vi "ParameterEditor_new.vi"(1 "Previous Parameters":T1=[{"Status"="ADC", "Name"="state (0,1,2)", "Value"=0.0, "Changed"=FALSE}, {"Status"="Camera", "Name"="state (0,1)", "Value"=0.0, "Changed"=FALSE}, {"Status"="Slave", "Name"="state (0,1)", "Value"=0.0, "Changed"=FALSE}, {"Status"="Wait", "Name"="inbit (0...7)", "Value"=0.0, "Changed"=FALSE}, {"Status"="e-", "Name"="enable (0,1)", "Value"=0.0, "Changed"=FALSE}, {"Status"="e-", "Name"="burn time (s)", "Value"=0.0, "Changed"=FALSE}, {"Status"="e-", "Name"="filament (A)", "Value"=0.0, "Changed"=FALSE}, {"Status"="RW", "Name"="enable (0,1)", "Value"=0.0, "Changed"=FALSE}, {"Status"="RW", "Name"="frequency (Hz)", "Value"=0.0, "Changed"=FALSE}, {"Status"="RW", "Name"="amplitude (V)", "Value"=0.0, "Changed"=FALSE}, {"Status"="RW", "Name"="d-phase (deg)", "Value"=0.0, "Changed"=FALSE}, {"Status"="HVpulse", "Name"="enable (0,1)", "Value"=0.0, "Changed"=FALSE}, {"Status"="HVpulse", "Name"="amplitude (V)", "Value"=0.0, "Changed"=FALSE}, {"Status"="HVpulse", "Name"="polarity (0=n)", "Value"=0.0, "Changed"=FALSE}, {"Status"="HVptime", "Name"="delay (s)", "Value"=0.0, "Changed"=FALSE}, {"Status"="HVptime", "Name"="width (s)", "Value"=0.0, "Changed"=FALSE}, {"Status"="Gcoil", "Name"="current (A)", "Value"=0.0, "Changed"=FALSE}, {"Status"="MCP", "Name"="front bias (V)", "Value"=0.0, "Changed"=FALSE}, {"Status"="MCP", "Name"="back bias (V)", "Value"=0.0, "Changed"=FALSE}, {"Status"="MCP", "Name"="phos bias (V)", "Value"=0.0, "Changed"=FALSE}] {"Value" format="%_6p"}, 2 "New Parameters":T1=[{"Status"="ADC", "Name"="state (0,1,2)", "Value"=0.0, "Changed"=FALSE}, {"Status"="Camera", "Name"="state (0,1)", "Value"=0.0, "Changed"=FALSE}, {"Status"="Slave", "Name"="state (0,1)", "Value"=0.0, "Changed"=FALSE}, {"Status"="Wait", "Name"="inbit (0...7)", "Value"=0.0, "Changed"=FALSE}, {"Status"="e-", "Name"="enable (0,1)", "Value"=0.0, "Changed"=FALSE}, {"Status"="e-", "Name"="burn time (s)", "Value"=0.0, "Changed"=FALSE}, {"Status"="e-", "Name"="filament (A)", "Value"=0.0, "Changed"=FALSE}, {"Status"="RW", "Name"="enable (0,1)", "Value"=0.0, "Changed"=FALSE}, {"Status"="RW", "Name"="frequency (Hz)", "Value"=0.0, "Changed"=FALSE}, {"Status"="RW", "Name"="amplitude (V)", "Value"=0.0, "Changed"=FALSE}, {"Status"="RW", "Name"="d-phase (deg)", "Value"=0.0, "Changed"=FALSE}, {"Status"="HVpulse", "Name"="enable (0,1)", "Value"=0.0, "Changed"=FALSE}, {"Status"="HVpulse", "Name"="amplitude (V)", "Value"=0.0, "Changed"=FALSE}, {"Status"="HVpulse", "Name"="polarity (0=n)", "Value"=0.0, "Changed"=FALSE}, {"Status"="HVptime", "Name"="delay (s)", "Value"=0.0, "Changed"=FALSE}, {"Status"="HVptime", "Name"="width (s)", "Value"=0.0, "Changed"=FALSE}, {"Status"="Gcoil", "Name"="current (A)", "Value"=0.0, "Changed"=FALSE}, {"Status"="MCP", "Name"="front bias (V)", "Value"=0.0, "Changed"=FALSE}, {"Status"="MCP", "Name"="back bias (V)", "Value"=0.0, "Changed"=FALSE}, {"Status"="MCP", "Name"="phos bias (V)", "Value"=0.0, "Changed"=FALSE}] {"Value" format="%_6p"}) -> (0 "Output parameters":T1=[{"Status"="ADC", "Name"="state (0,1,2)", "Value"=0.0, "Changed"=FALSE}, {"Status"="Camera", "Name"="state (0,1)", "Value"=0.0, "Changed"=FALSE}, {"Status"="Slave", "Name"="state (0,1)", "Value"=0.0, "Changed"=FALSE}, {"Status"="Wait", "Name"="inbit (0...7)", "Value"=0.0, "Changed"=FALSE}, {"Status"="e-", "Name"="enable (0,1)", "Value"=0.0, "Changed"=FALSE}, {"Status"="e-", "Name"="burn time (s)", "Value"=0.0, "Changed"=FALSE}, {"Status"="e-", "Name"="filament (A)", "Value"=0.0, "Changed"=FALSE}, {"Status"="RW", "Name"="enable (0,1)", "Value"=0.0, "Changed"=FALSE}, {"Status"="RW", "Name"="frequency (Hz)", "Value"=0.0, "Changed"=FALSE}, {"Status"="RW", "Name"="amplitude (V)", "Value"=0.0, "Changed"=FALSE}, {"Status"="RW", "Name"="d-phase (deg)", "Value"=0.0, "Changed"=FALSE}, {"Status"="HVpulse", "Name"="enable (0,1)", "Value"=0.0, "Changed"=FALSE}, {"Status"="HVpulse", "Name"="amplitude (V)", "Value"=0.0, "Changed"=FALSE}, {"Status"="HVpulse", "Name"="polarity (0=n)", "Value"=0.0, "Changed"=FALSE}, {"Status"="HVptime", "Name"="delay (s)", "Value"=0.0, "Changed"=FALSE}, {"Status"="HVptime", "Name"="width (s)", "Value"=0.0, "Changed"=FALSE}, {"Status"="Gcoil", "Name"="current (A)", "Value"=0.0, "Changed"=FALSE}, {"Status"="MCP", "Name"="front bias (V)", "Value"=0.0, "Changed"=FALSE}, {"Status"="MCP", "Name"="back bias (V)", "Value"=0.0, "Changed"=FALSE}, {"Status"="MCP", "Name"="phos bias (V)", "Value"=0.0, "Changed"=FALSE}] {"Value" format="%_6p"})   [LabVIEW 2018]
uses:
  Parameters.ctl
panel:
  in  "Load previous":bool
  in  "Done":bool
  in  "Parameter History":enum32{"New", "Previous", "Output"}(tab)
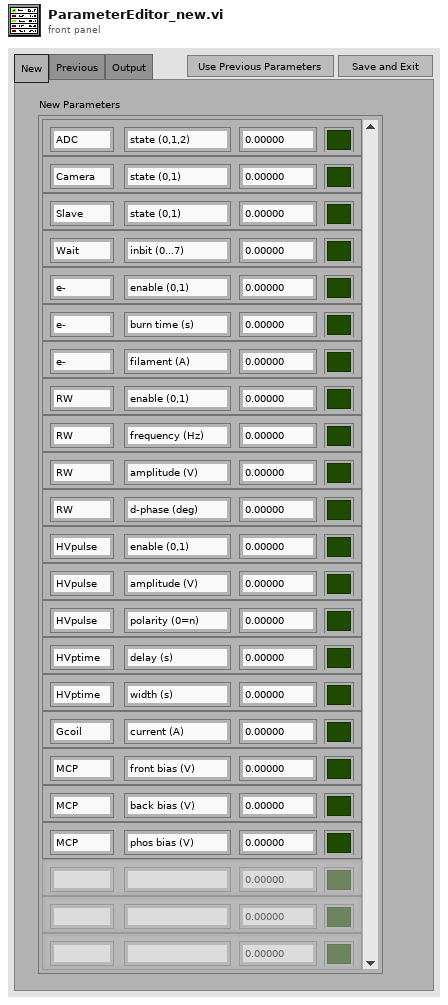
[diagram p1: front panel]
types:
  T1 = typedef "Parameters.ctl" = cluster{"Status":string, "Name":string, "Value":dbl, "Changed":bool}[]
  T2 = cluster{"Status":string, "Name":string, "Value":dbl, "Changed":bool}
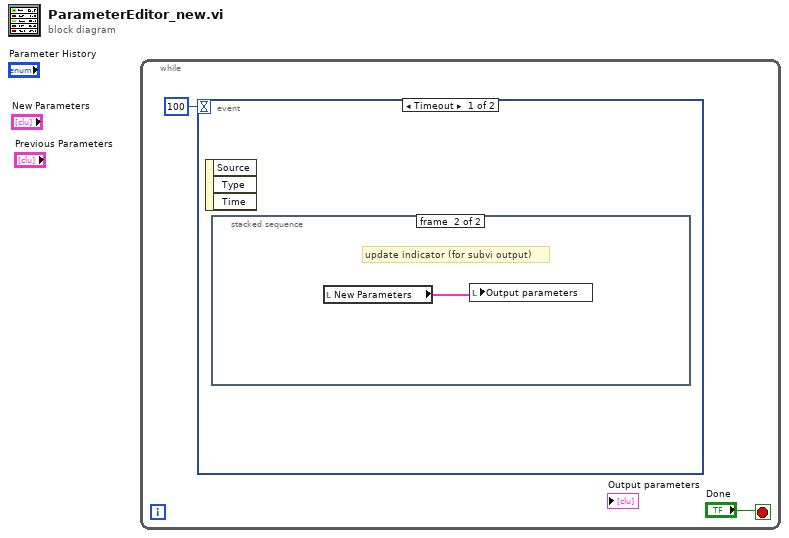
[diagram p0: block diagram]
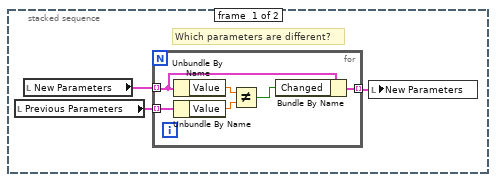
[diagram p2: hidden frame]
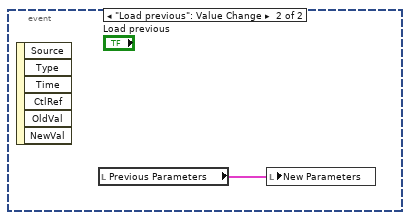
[diagram p3: hidden frame]
diagram:
  n1 = while {
    stop <- "Done" stop-if-true
    n2 = event shown="[0] Timeout" {
      selector: _ -> [_ _]
      dyn-events: _ -> [_ _]
      timeout: 100 -> [_ _]
      event Timeout {
        n3 = event-data() -> ()  [unwired: 1 in, 3 out]
        n4 = stacked-sequence {
          frame #0 {
            # "Which parameters are different?"
            n5 = local read "Previous Parameters"() -> (w5:T1)
            n6 = local read "New Parameters"() -> (w4:T1)
            n7 = for {
              tunnel: w4 -> [w8] mode=indexing
              tunnel: w5 -> [w11] mode=indexing
              tunnel: [w6] -> w3 mode=indexing
              n8 = Unbundle By Name(w8) -> ("Value"=w10:dbl)
              n9 = Unbundle By Name(w11) -> ("Value"=w9:dbl)
              n10 = Not Equal?(x=w10, y=w9) -> (x != y?=w7:bool)
              n11 = Bundle By Name(cluster=w8, "Changed"=w7) -> (w6:T2)
            }
            n12 = local write "New Parameters"(w3) -> ()
          }
          frame #1 {
            # "update indicator (for subvi output)"
            n13 = local read "New Parameters"() -> (w12:T1)
            n14 = local write "Output parameters"(w12) -> ()
          }
        }
      }
      event "Load previous": Value Change {
        n15 = event-data() -> ()  [unwired: 1 in, 6 out]
        n16 = local read "Previous Parameters"() -> (w13:T1)
        n17 = local write "New Parameters"(w13) -> ()
      }
    }
  }
